vi "Measurement.PhotocurrentMapping.DVRtoRef.vi"(10 "Ref":T1) -> (2 "Ref":u32 format="%08x")   [LabVIEW 2017, in "Measurement.PhotocurrentMapping.lvclass"]
doc: "JKI State Machine Objects (SMO) 1.0.0.5\nJKI - JKI\nCopyright (c) 2016, JKI"
uses:
  Measurement.PhotocurrentMapping.lvclass
  Typedefs/PrivateData--Ref.ctl
  Typedefs/PrivateData--Cluster.ctl
  Typedefs/Configuration--Cluster.ctl
  Measurement/Typedefs/Measurement.Type--Enum.ctl
  Typedefs/Configuration.Hardware--Cluster.ctl
  Measurement/Typedefs/Configuration.SMU--Cluster.ctl
  SMU/Typedefs/Configuration--Cluster.ctl
  Measurement/Typedefs/Configuration.LIA--Cluster.ctl
  LIA/Typedefs/Configuration--Cluster.ctl
  Measurement/Typedefs/Configuration.XYStage--Cluster.ctl
  XYStage/Typedefs/Configuration--Cluster.ctl
  Typedefs/Configuration.Measurement--Cluster.ctl
  Typedefs/Configuration.Axis--Cluster.ctl
  Typedefs/Dependencies--Cluster.ctl
  SMU/SMU.lvclass
  LIA/LIA.lvclass
  XYStage/XYStage.lvclass
  Measurement/Measurement.lvclass
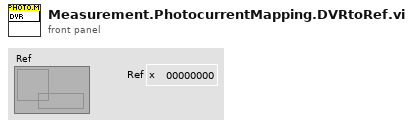
[diagram p1: front panel]
types:
  T1 = typedef "Measurement.PhotocurrentMapping.lvclass/PrivateData--Ref.ctl" = refnum<data-value>
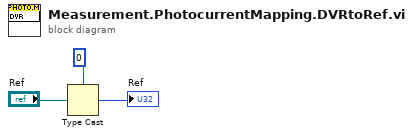
[diagram p0: block diagram]
diagram:
  n1 = Type Cast(type=u32 0 ("Ref"), x="Ref") -> (*(type *) &x=→"Ref":u32)
